vi "TCP-Quit Server.vi"(7 "Name":string) -> (15 "error out":errorcluster)   [LabVIEW 2020]
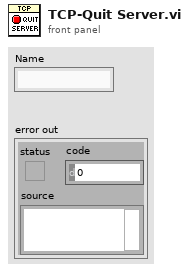
[diagram p1: front panel]
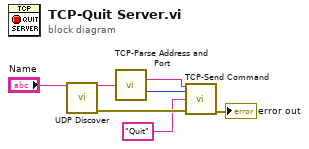
[diagram p0: block diagram]
diagram:
  n1 = call "UDP Discover.vi"("Name"="Name") -> ("address:port"=w3:string, "error out"=w7:errorcluster)  [unwired: 9 in, 4 out]
  n2 = call "TCP-Parse Address and Port.vi"("Address in"=w3) -> ("Address"=w2:string, "Port"=w1:i32)  [unwired: 12 in, 1 out]
  n3 = call "TCP-Send Command.vi"("PXI Address"=w2, "Port"=w1, "Command"="Quit", "error in (no error)"=w7) -> ("error out"=→"error out":errorcluster)  [unwired: 11 in]
